vi "Autosize Listbox Columns (Uniform Text).vi"(4 "error in (no error)":errorcluster, 5 "extra padding (0)":i16, 6 "Resize Table? (F)":bool, 7 "Table Ref":refnum<vi>) -> (0 "error out":errorcluster, 3 "Table Ref":refnum<vi>)   [LabVIEW 2019, in "MutationHistoryGUI.lvlib"]
doc: "This VI resizes each column of the table specified by Table Ref based on the widest entry of the column. Additionally, if Resize Table? is TRUE, the VI will set the table width based on the number of populated columns."
uses:
  MutationHistoryGUI.lvlib
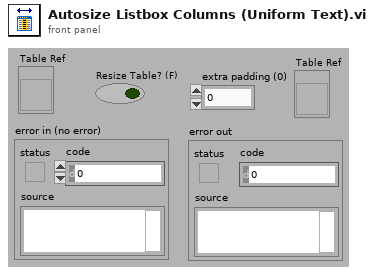
[diagram p1: front panel]
types:
  T1 = enum16{"User-specified Font", "Application Font", "System Font", "Dialog Font"}
  T2 = cluster{"Font Name:":string, "Size":i16, "Strikeout?":bool, "Italic?":bool, "Underline?":bool, "Outline?":bool, "Shadow?":bool, "Bold?":bool}
  T3 = cluster{"left":i16, "top":i16, "right":i16, "bottom":i16}
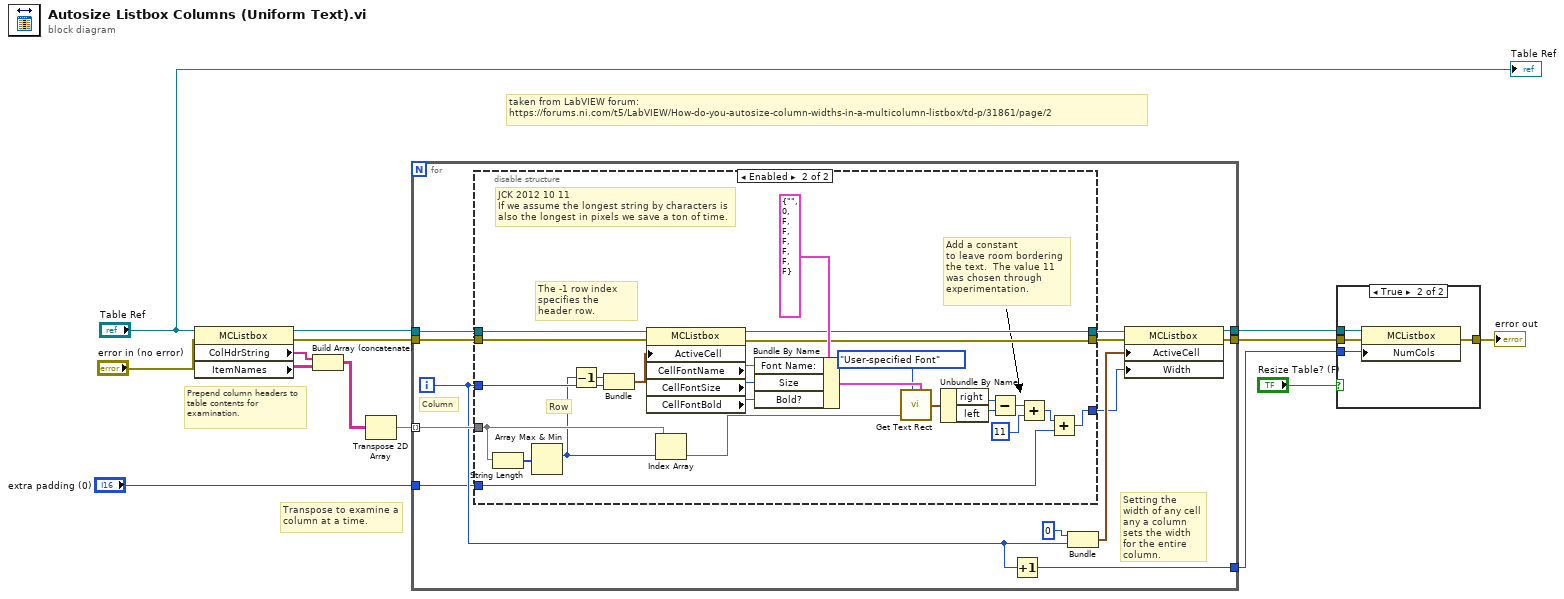
[diagram p0: block diagram]
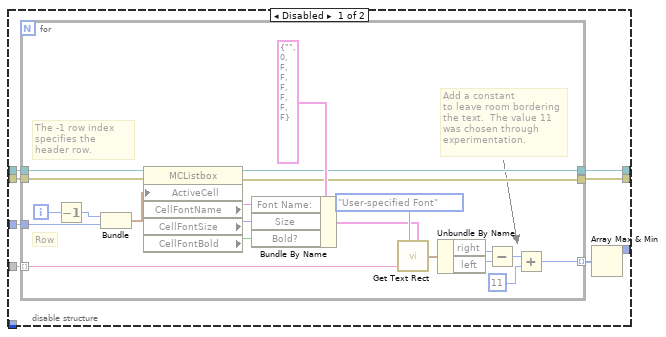
[diagram p3: hidden frame]
diagram:
  # "taken from LabVIEW forum:\nhttps://forums.ni.com/t5/LabVIEW/How-do-you-autosize-column-widths-in-a-multicolumn-listbox/td-p/31861/page/2"
  # "Transpose to examine a column at a time."
  # "Prepend column headers to table contents for examination."
  n1 = property class="MCListbox"(reference="Table Ref", error in="error in (no error)") -> (reference out=w14:refnum<vi>, error out=w10:errorcluster, "ColHdrString"=w13:string[], "ItemNames"=w9:string[][])
  n2 = Build Array (concatenate)(w13, w9) -> (w12:string[][])
  n3 = Transpose 2D Array(2D array=w12) -> (transposed array=w11:string[][])
  n4 = for {
    tunnel: w11 -> [w27] mode=indexing
    tunnel: w14 -> [w26]
    tunnel: w10 -> [w25]
    tunnel: [w19] -> w5
    tunnel: [w18] -> w6
    tunnel: [w16] -> w4
    tunnel: "extra padding (0)" -> [w15]
    i -> [w17]
    # "Setting the width of any cell any a column sets the width for the entire column."
    # "Column"
    n5 = disable-structure shown="Enabled" {
      disable-tunnel: w27 -> [w35 w66]
      disable-tunnel: w26 -> [w34 w63]
      disable-tunnel: w25 -> [w32 w62]
      disable-tunnel: [w31 w61] -> w24
      disable-tunnel: [w30 w60] -> w23
      disable-tunnel: [w29 w58] -> w20
      disable-tunnel: w17 -> [w28 w67]
      disable-tunnel: w15 -> [_ w57]
      frame Disabled {
        n6 = for {
          tunnel: w35 -> [w48] mode=indexing
          tunnel: w34 -> [w56]
          tunnel: w28 -> [w55]
          tunnel: [w37] -> w33 mode=indexing
          tunnel: w32 -> [w42]
          tunnel: [w41] -> w30
          tunnel: [w40] -> w31
          i -> [w44]
          # "The -1 row index specifies the header row."
          # "Add a constant\nto leave room bordering the text.  The value 11 was chosen through experimentation."
          # "Row"
          n7 = Decrement(x=w44) -> (x-1=w43:i32)
          n8 = Bundle(w43, w55) -> (w54:cluster{i32, i32})  [unwired: 1 in]
          n9 = property class="MCListbox"(reference=w56, error in=w42, "ActiveCell"=w54) -> (reference out=w40:refnum<vi>, error out=w41:errorcluster, "CellFontName"=w52:string, "CellFontSize"=w38:u32, "CellFontBold"=w51:bool)
          n10 = Bundle By Name(cluster=T2 {"Font Name:"="", "Size"=0, "Strikeout?"=FALSE, "Italic?"=FALSE, "Underline?"=FALSE, "Outline?"=FALSE, "Shadow?"=FALSE, "Bold?"=FALSE} ("[user-specified font]"), "Font Name:"=w52, "Size"=w38, "Bold?"=w51) -> (w49:T2)
          n11 = call <vilib>:"Get Text Rect.vi"("desired font(Application)"=T1."User-specified Font", "text"=w48, "[user-specified font]"=w49) -> ("rect"=w47:T3)  [unwired: 6 in]
          n12 = Unbundle By Name(w47) -> ("right"=w46:i16, "left"=w45:i16)
          n13 = Subtract(x=w46, y=w45) -> (x-y=w39:i16)
          n14 = Add(x=w39, y=i16 11) -> (x+y=w37:i16)
        }
        n15 = Array Max & Min(array=w33) -> (max value=w29:i16)  [unwired: 3 out]
      }
      frame Enabled {
        # "JCK 2012 10 11\nIf we assume the longest string by characters is also the longest in pixels we save a ton of time."
        # "The -1 row index specifies the header row."
        # "Add a constant\nto leave room bordering the text.  The value 11 was chosen through experimentation."
        # "Row"
        n16 = String Length(string=w66) -> (length=w81:i32[])
        n17 = Array Max & Min(array=w81) -> (max index (indices)=w65:i32)  [unwired: 3 out]
        n18 = Decrement(x=w65) -> (x-1=w77:i32)
        n19 = Bundle(w77, w67) -> (w68:cluster{i32, i32})  [unwired: 1 in]
        n20 = property class="MCListbox"(reference=w63, error in=w62, "ActiveCell"=w68) -> (reference out=w61:refnum<vi>, error out=w60:errorcluster, "CellFontName"=w70:string, "CellFontSize"=w79:u32, "CellFontBold"=w71:bool)
        n21 = Index Array(array=w66, index=w65) -> (element=w64:string)
        n22 = Bundle By Name(cluster=T2 {"Font Name:"="", "Size"=0, "Strikeout?"=FALSE, "Italic?"=FALSE, "Underline?"=FALSE, "Outline?"=FALSE, "Shadow?"=FALSE, "Bold?"=FALSE} ("[user-specified font]"), "Font Name:"=w70, "Size"=w79, "Bold?"=w71) -> (w73:T2)
        n23 = call <vilib>:"Get Text Rect.vi"("desired font(Application)"=T1."User-specified Font", "text"=w64, "[user-specified font]"=w73) -> ("rect"=w74:T3)  [unwired: 6 in]
        n24 = Unbundle By Name(w74) -> ("right"=w75:i16, "left"=w76:i16)
        n25 = Subtract(x=w75, y=w76) -> (x-y=w78:i16)
        n26 = Add(x=w78, y=i16 11) -> (x+y=w59:i16)
        n27 = Add(x=w59, y=w57) -> (x+y=w58:i16)
      }
    }
    n28 = Increment(x=w17) -> (x+1=w16:i32)
    n29 = Bundle(0, w17) -> (w21:cluster{i32, i32})  [unwired: 1 in]
    n30 = property class="MCListbox"(reference=w24, error in=w23, "ActiveCell"=w21, "Width"=w20) -> (reference out=w18:refnum<vi>, error out=w19:errorcluster)
  }
  n31 = case shown="True" "Resize Table? (F)" {
    tunnel: w6 -> [_ w86]
    tunnel: w5 -> [w82 w85]
    tunnel: w4 -> [_ w84]
    tunnel: [w82 w83] -> w3
    frame False {
    }
    frame True {
      n32 = property class="MCListbox"(reference=w86, error in=w85, "NumCols"=w84) -> (error out=w83:errorcluster)  [unwired: 1 out]
    }
  }
  "error out" <- w3
  "Table Ref" <- "Table Ref"
